vi "SlewRateLimiter_GetRate.vi"(11 "in SLEW_RATE_LIMITER":T1 {"Timer"."Accumulated TIme" format="%13.5p"; "Timer"."StartTime" format="%13.5p"; "PrevValue" format="%13.5p"; "RateLimit" format="%13.5p"}) -> (3 "Rate":dbl)   [LabVIEW 2019, in "Trajectory_Library.lvlib"]
doc: "Gets the current rate limit value.\n\nInputs:\n - in Slew Rate Limiter -- The Slew Rate Limiter data cluster\n \nOutputs:\n - rate -- The current rate limit in units/second."
uses:
  Trajectory_Library.lvlib
  SLEW_RATE_LIMITER.ctl
  TIMER.ctl
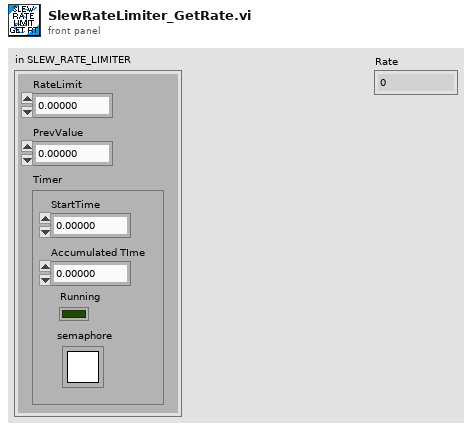
[diagram p1: front panel]
types:
  T1 = typedef "Trajectory_Library.lvlib/SLEW_RATE_LIMITER.ctl" = cluster{"RateLimit":dbl, "PrevValue":dbl, "Timer":T2}
  T2 = typedef "Trajectory_Library.lvlib/TIMER.ctl" = cluster{"StartTime":dbl, "Accumulated TIme":dbl, "Running":bool, "semaphore":T3}
  T3 = typedef "Semaphore RefNum" = refnum<k1>
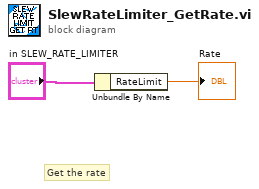
[diagram p0: block diagram]
diagram:
  # "Get the rate"
  n1 = Unbundle By Name("in SLEW_RATE_LIMITER") -> ("RateLimit"=→"Rate":dbl)
